vi "Query Remote Sense State.vi"(8 "error in (no error)":errorcluster, 11 "VISA resource name":refnum<visa-resource-name>) -> (0 "error out":errorcluster, 2 "Remote Sense Enabled":bool, 3 "VISA resource name out":refnum<visa-resource-name>)   [LabVIEW 2018, in "XP Power PLS600.lvlib"]
doc: "Queries the present remote sense state of the power supply. True indicates remote sense is on or active, False indicates that it is off or deactive."
uses:
  XP Power PLS600.lvlib
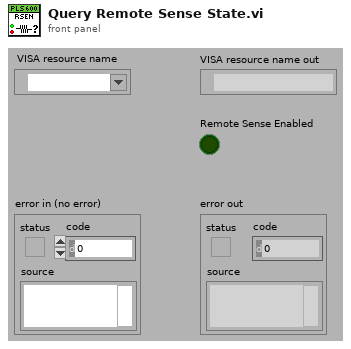
[diagram p1: front panel]
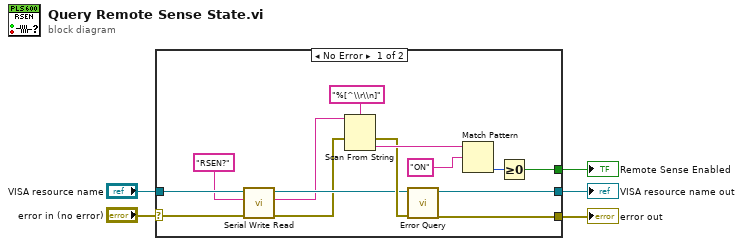
[diagram p0: block diagram]
diagram:
  n1 = case shown="No Error" "error in (no error)" {
    selector: "error in (no error)" -> [w6 w21]
    tunnel: [w19 w20] -> w5
    tunnel: [w18 w21] -> w4
    tunnel: [w13 _] -> w3
    tunnel: "VISA resource name" -> [w11 w20]
    frame No Error {
      n2 = call "Serial Write Read.vi"("error in (no error)"=w6, "Write Buffer"="RSEN?", "VISA resource name"=w11) -> ("error out"=w7:errorcluster, "Read Buffer"=w8:string, "VISA resource name out"=w9:refnum<visa-resource-name>)  [unwired: 6 in]
      n3 = Scan From String(format string="%[^\\r\\n]", input string=w8, error in=w7) -> (error out=w12:errorcluster, output 1=w16:string)  [unwired: 2 in, 2 out]
      n4 = call "Error Query.vi"("error in (no error)"=w12, "VISA resource name"=w9) -> ("error out"=w18:errorcluster, "VISA resource name out"=w19:refnum<visa-resource-name>)  [unwired: 6 in, 2 out]
      n5 = Match Pattern(string=w16, regular expression="ON" ("y")) -> (offset past match=w14:i32)  [unwired: 1 in, 3 out]
      n6 = Greater Or Equal To 0?(x=w14) -> (x >= 0?=w13:bool)
    }
    frame Error {
    }
  }
  "VISA resource name out" <- w5
  "error out" <- w4
  "Remote Sense Enabled" <- w3
